vi "Read AxisNumber.vi"(8 "error in (no error)":errorcluster, 11 "Picomotor8742Axis in":refnum<class "Picomotor8742Axis.lvclass">) -> (0 "error out":errorcluster, 2 "AxisNumber":i32, 3 "Picomotor8742Axis out":refnum<class "Picomotor8742Axis.lvclass">)   [LabVIEW 2020, in "Picomotor8742Axis.lvclass"]
uses:
  Picomotor8742Axis.lvclass
  Picomotor8742Axis.lvclass/Picomotor8742Axis.ctl
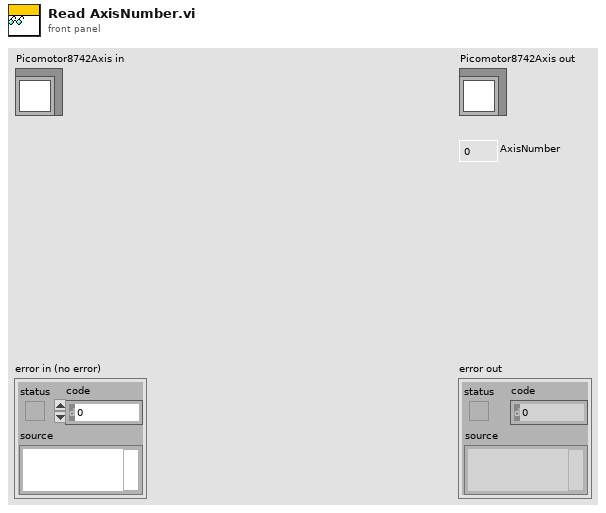
[diagram p1: front panel]
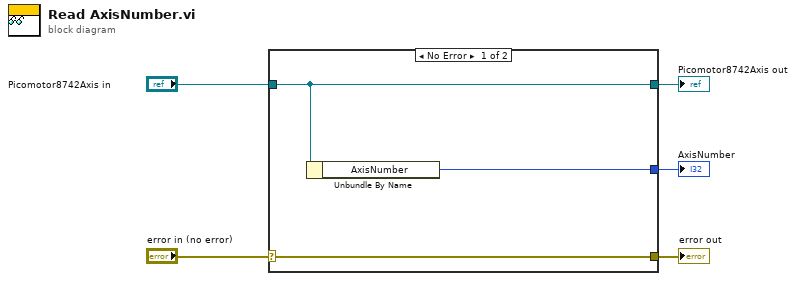
[diagram p0: block diagram]
diagram:
  n1 = case shown="No Error" "error in (no error)" {
    selector: "error in (no error)" -> [w8 w9]
    tunnel: [w8 w9] -> w4
    tunnel: [w7 w10] -> w2
    tunnel: "Picomotor8742Axis in" -> [w7 w10]
    tunnel: [w6 _] -> w1
    frame No Error {
      n2 = Unbundle By Name(w7) -> ("AxisNumber"=w6:i32)
    }
    frame Error {
    }
  }
  "error out" <- w4
  "Picomotor8742Axis out" <- w2
  "AxisNumber" <- w1
